vi "SQL_table_load_insert.vi"(0 "testId":string, 1 "供油油温":dbl, 2 "供油流量":dbl, 7 "转速":dbl, 9 "轴向载荷":dbl, 11 "径向载荷":dbl, 12 "供油压力":dbl, 13 "持续时间":dbl, 14 "结果":string) -> (4 "error out":errorcluster)   [LabVIEW 2014]
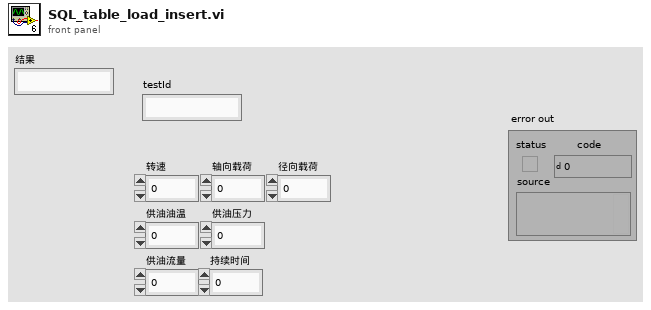
[diagram p1: front panel]
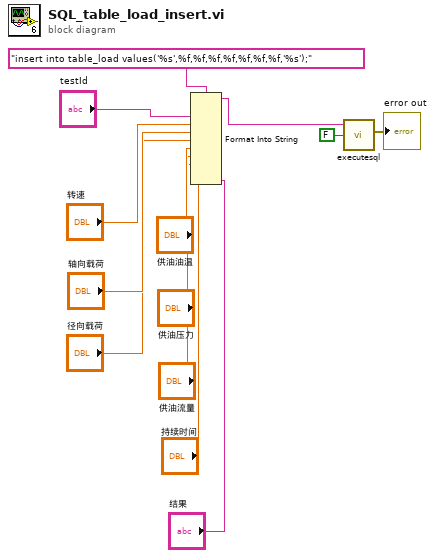
[diagram p0: block diagram]
diagram:
  n1 = Format Into String(format string="insert into table_load values('%s',%f,%f,%f,%f,%f,%f,%f,'%s');" ("Command Text"), "testId", "转速", "轴向载荷", "径向载荷", "供油油温", "供油压力", "供油流量", "持续时间", "结果") -> (resulting string=w5:string)  [unwired: 2 in, 1 out]
  n2 = call "executesql.vi"("Return Data (T)"=FALSE, "Command Text"=w5) -> ("error out"=→"error out":errorcluster)  [unwired: 5 in, 1 out]
